vi "AnalyzePatternMatches (SubVI).vi"(6 "Match position variation tolerance":sgl, 7 "Image in":T1, 8 "true y":sgl=1496.0, 9 "true x":sgl=313.0, 10 "Number of Matches":i32, 11 "Matches (pixel)":T2(array[cluster])) -> (1 "True Match Index":i32, 2 "True Match Score":sgl, 3 "Display with box":T1, 5 "Image out":T1)   [LabVIEW 2016]
uses:
  <vilib>/vision/Image Controls.llb/IMAQ Image.ctl
panel:
  # "Purpose of this subVI is to:\n- Draw boxes around all pattern matches\nidentified in image\n- Identify the \"true match\" based on its coordinates\nand output the true match's score"
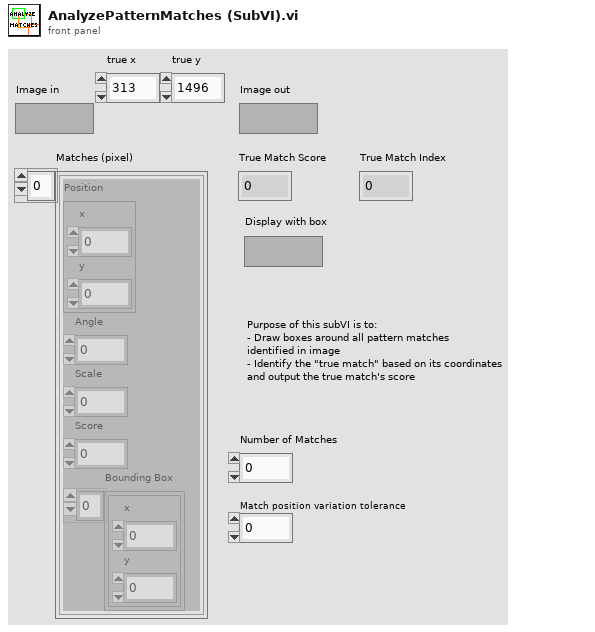
[diagram p1: front panel]
types:
  T1 = typedef "IMAQ Image.ctl" = refnum<image>
  T2 = cluster{"Position":cluster{"x":sgl, "y":sgl}, "Angle":sgl, "Scale":sgl, "Score":sgl, "Bounding Box":cluster{"x":sgl, "y":sgl}[]}[]
  T3 = cluster{"Position":cluster{"x":sgl, "y":sgl}, "Angle":sgl, "Scale":sgl, "Score":sgl, "Bounding Box":cluster{"x":sgl, "y":sgl}[]}
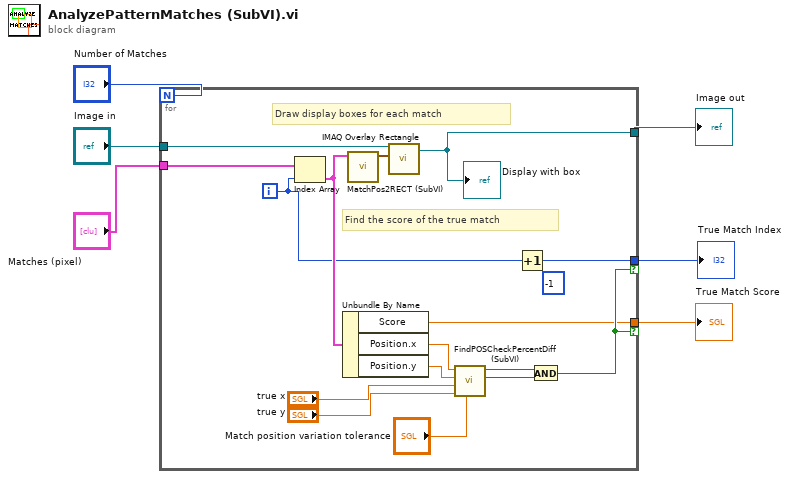
[diagram p0: block diagram]
diagram:
  n1 = for {
    N: "Number of Matches" -> [_]
    tunnel: "Matches (pixel)" -> [w22]
    tunnel: [w20] -> w4
    tunnel: "Image in" -> [w19]
    tunnel: [w9] -> w6 if=w10
    tunnel: [w8] -> w1 if=w10
    i -> [w7]
    (unwired) -1
    # "Draw display boxes for each match"
    # "Find the score of the true match"
    n2 = Index Array(array=w22, index=w7) -> (element=w18:T3)
    n3 = Unbundle By Name(w18) -> ("Score"=w9:sgl, "Position.x"=w17:sgl, "Position.y"=w16:sgl)
    n4 = call "MatchPos2RECT (SubVI).vi"("Match element"=w18) -> ("Rectangle"=w21:cluster{"x":sgl, "y":sgl, dbl, dbl})  [unwired: 10 in]
    n5 = call "IMAQ Overlay Rectangle"("Rectangle"=w21, "Image"=w19) -> ("Image Out"=w20:T1)  [unwired: 8 in, 1 out]
    "Display with box" <- w20
    n6 = call "FindPOSCheckPercentDiff (SubVI).vi"("x"=w17, "y"=w16, "true x"="true x", "true y"="true y", "variation tolerance"="Match position variation tolerance") -> ("pass x coordinate"=w12:bool, "pass y coordinate"=w11:bool)  [unwired: 4 in]
    n7 = Increment(x=w7) -> (x+1=w8:i32)
    n8 = And(x=w12, y=w11) -> (x .and. y?=w10:bool)
  }
  "True Match Score" <- w6
  "Image out" <- w4
  "True Match Index" <- w1
